vi "Deferer.vi"(8 "error in (no error)":errorcluster) -> (0 "error out":errorcluster, 3 "Deferer out":refnum<class "Deferer.lvclass">)   [LabVIEW 2019, in "Panel.lvlib" / "Deferer.lvclass"]
doc: "Creates a new defer instance.\n\n----\nPlease see the following web address for additional documentation and tutorial information:\nhttp://www.mooregoodideas.com/mgi-panel-manager/\n\nAuthor: Derek Trepanier\n\nCopyright (c) 2018, Moore Good Ideas, Inc.\n\nAll rights reserved.\n\nRedistribution and use in source and binary forms, with or without modification, are permitted provided that the following conditions are met:\n\n * Redistributions of source code must retain the above copyright notice, this list of conditions and the following disclaimer.\n * Redistributions in binary form must reproduce the above copyright notice, this list of conditions and the following disclaimer in the documentation and/or other materials provided with the distribution.\n * Neither the name of Moore Good Ideas, Inc. nor the names of its contributors may be used to endorse or promote products derived from this software without specific prior written permission.\n\nTHIS SOFTWARE IS PROVIDED BY THE COPYRIGHT HOLDERS AND CONTRIBUTORS \"AS IS\" AND ANY EXPRESS OR IMPLIED WARRANTIES, INCLUDING, BUT NOT LIMITED TO, THE IMPLIED WARRANTIES OF MERCHANTABILITY AND FITNESS FOR A PARTICULAR PURPOSE ARE DISCLAIMED. IN NO EVENT SHALL THE COPYRIGHT OWNER OR CONTRIBUTORS BE LIABLE FOR ANY DIRECT, INDIRECT, INCIDENTAL, SPECIAL, EXEMPLARY, OR CONSEQUENTIAL DAMAGES (INCLUDING, BUT NOT LIMITED TO, PROCUREMENT OF SUBSTITUTE GOODS OR SERVICES; LOSS OF USE, DATA, OR PROFITS; OR BUSINESS INTERRUPTION) HOWEVER CAUSED AND ON ANY THEORY OF LIABILITY, WHETHER IN CONTRACT, STRICT LIABILITY, OR TORT (INCLUDING NEGLIGENCE OR OTHERWISE) ARISING IN ANY WAY OUT OF THE USE OF THIS SOFTWARE, EVEN IF ADVISED OF THE POSSIBILITY OF SUCH DAMAGE."
uses:
  Deferer.lvclass
  Deferer.lvclass/Deferer.ctl
  Panel Control Counter/Panel Control Counter.lvclass
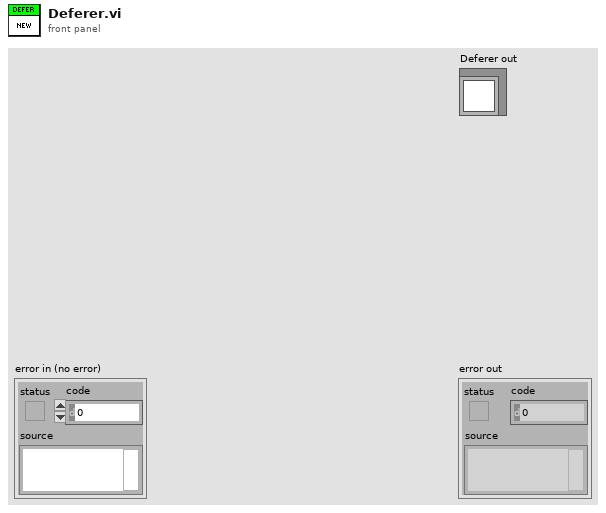
[diagram p1: front panel]
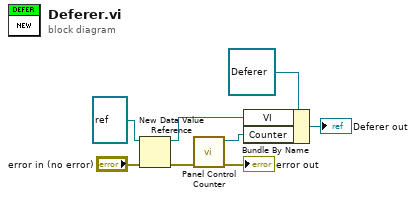
[diagram p0: block diagram]
diagram:
  n1 = New Data Value Reference(data value=refnum<vi> refnum ("VI"), error in="error in (no error)") -> (data value reference=w4:refnum<data-value>, error out=w3:errorcluster)
  n2 = call "Panel Control Counter.vi"("error in (no error)"=w3) -> ("error out"=→"error out":errorcluster, "Panel Control Counter out"=w1:refnum<class "Panel Control Counter.lvclass">)  [unwired: 9 in]
  n3 = Bundle By Name(cluster=refnum<class "Deferer.lvclass"> refnum ("Deferer in"), "VI"=w4, "Counter"=w1) -> (→"Deferer out":refnum<class "Deferer.lvclass">)
